vi "Read pubDataEvents.vi"(11 "PubSubDataEvent in":refnum<class "PubSubDataEvent.lvclass">) -> (2 "pubDataEvents":T1, 3 "PubSubDataEvent out":refnum<class "PubSubDataEvent.lvclass">)   [LabVIEW 2016, in "PubSubDataEvent.lvclass"]
uses:
  PubSubDataEvent.lvclass
  TypedefsDataEvents/PubDataEvents.ctl
  ts_sallv_exa/DataTypes/logevent_SettingVersions.ctl
  ts_sallv_exa/DataTypes/logevent_SummaryState.ctl
  ts_sallv_exa/DataTypes/logevent_RejectedCommand.ctl
  ts_sallv_exa/DataTypes/logevent_DetailedState.ctl
  ts_sallv_exa/DataTypes/logevent_ErrorCode.ctl
  ts_sallv_exa/DataTypes/logevent_Heartbeat.ctl
  ts_sallv_exa/DataTypes/LoopTime_ms.ctl
  ts_sallv_exa/DataTypes/logevent_LoopTimeOutOfRange.ctl
  ts_sallv_exa/DataTypes/Timestamp.ctl
  PubSubDataEvent.lvclass/PubSubDataEvent.ctl
  ts_sallv_exa/SALLV_EXA.lvlib
  TypedefsDataEvents/TypedefsDataEvents.lvlib
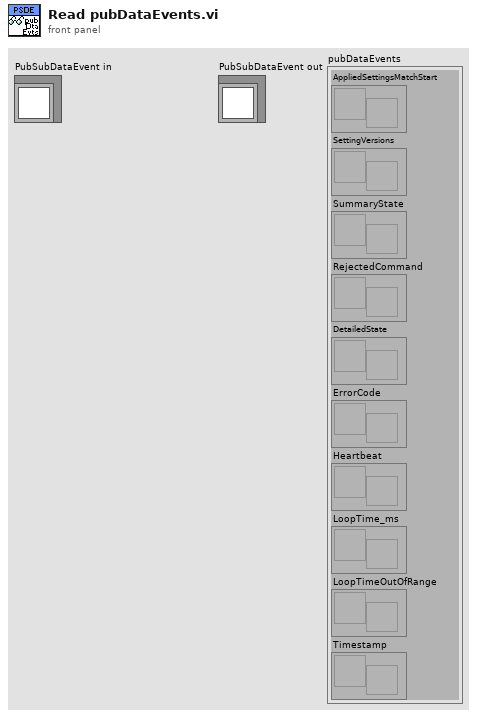
[diagram p1: front panel]
types:
  T1 = typedef "TypedefsDataEvents.lvlib/PubDataEvents.ctl" = cluster{"AppliedSettingsMatchStart":refnum<user-event>, "SettingVersions":refnum<user-event>, "SummaryState":refnum<user-event>, "RejectedCommand":refnum<user-event>, "DetailedState":refnum<user-event>, "ErrorCode":refnum<user-event>, "Heartbeat":refnum<user-event>, "LoopTime_ms":refnum<user-event>, "LoopTimeOutOfRange":refnum<user-event>, "Timestamp":refnum<user-event>}
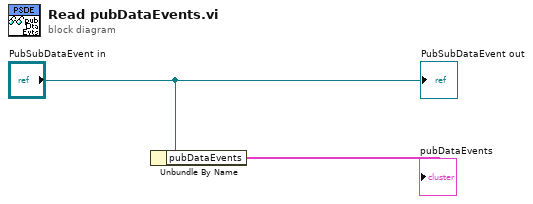
[diagram p0: block diagram]
diagram:
  n1 = Unbundle By Name("PubSubDataEvent in") -> ("pubDataEvents"=→"pubDataEvents":T1)
  "PubSubDataEvent out" <- "PubSubDataEvent in"
